vi "Instrument Do Core.vi"(8 "error in (no error)":errorcluster, 9 "Instrument in":refnum<class "Instrument Driver.lvclass">, 10 "Actor in":refnum<class "Actor.lvclass">, 11 "DMM Config Msg in":refnum<class "DMM List Triggers Msg.lvclass">) -> (0 "error out":errorcluster, 1 "Instrument out":refnum<class "Instrument Driver.lvclass">, 2 "Actor out":refnum<class "Actor.lvclass">, 3 "DMM Config Msg out":refnum<class "DMM List Triggers Msg.lvclass">, 5 "Data":refnum<class "Data.lvclass">)   [LabVIEW 2020, in "DMM Msg.lvlib" / "DMM List Triggers Msg.lvclass"]
doc: "List the triggers supported by the DMM Driver and return their names in a generic String Array class."
uses:
  DMM List Triggers Msg.lvclass
  PPL/HDH.Actor Framework.Core.Actor.lvlibp/1abvi3w/vi.lib/ActorFramework/Actor/Actor.lvclass
  PPL/HDH.Data.Generic.lvlibp/Data.lvclass
  PPL/HDH.Actor Framework.Core.Instrument Driver.lvlibp/Instrument Driver/Instrument Driver.lvclass
  PPL/HDH.Driver.DMM.lvlibp/DMM Driver.lvclass
  C:/Current projects/WS/PPL/HDH.Actor Framework.Core.Instrument Driver.lvlibp/Instrument Driver/Instrument Driver.lvclass
  PPL/HDH.Data.Generic.lvlibp/Generic Data/Generic Array Data/String Array/String Array.lvclass
  C:/Current projects/WS/PPL/HDH.Data.Generic.lvlibp/Data.lvclass
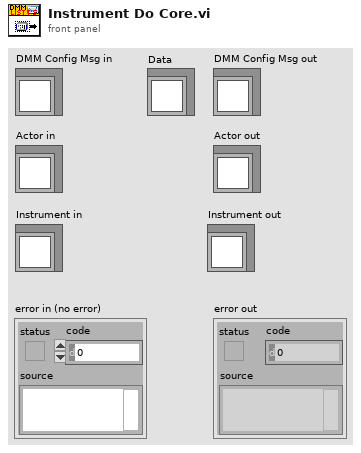
[diagram p1: front panel]
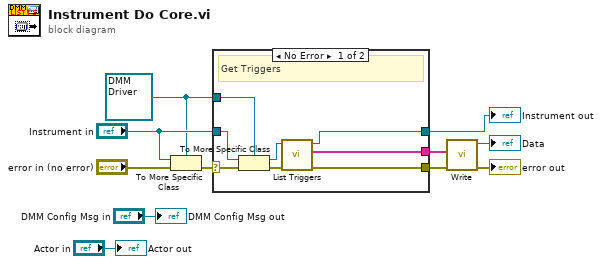
[diagram p0: block diagram]
diagram:
  w6 = refnum<class "DMM Driver.lvclass"> refnum ("HDH.Driver.DMM.lvlibp:DMM Driver.lvclass")
  n1 = To More Specific Class(target class=w6, reference="Instrument in", error in="error in (no error)") -> (error out=w9:errorcluster)  [unwired: 1 out]
  n2 = case shown="No Error" w9 {
    selector: w9 -> [w18 w20]
    tunnel: [w13 w20] -> w1
    tunnel: [w12 w19] -> w8
    tunnel: "Instrument in" -> [w17 w19]
    tunnel: w6 -> [w16 _]
    tunnel: [w11 _] -> w2
    frame No Error {
      # "Get Triggers"
      n3 = To More Specific Class(target class=w16, reference=w17, error in=w18) -> (specific class reference=w15:refnum<class "DMM Driver.lvclass">, error out=w14:errorcluster)
      n4 = call-dynamic "List Triggers.vi"("error in (no error)"=w14, "DMM Driver in"=w15) -> ("error out"=w13:errorcluster, "Trigger Names"=w11:string[], "DMM Driver out"=w12:refnum<class "DMM Driver.lvclass">)  [unwired: 7 in]
    }
    frame Error {
      # "Incorrect instrument - Return error"
    }
  }
  "error out" <- w1
  "Instrument out" <- w8
  n5 = call "Write.vi"("String Array"=w2) -> ("String Array out"=→"Data":refnum<class "String Array.lvclass">)  [unwired: 10 in]
  "DMM Config Msg out" <- "DMM Config Msg in"
  "Actor out" <- "Actor in"
